vi "CalGas Filtern - Elemente ermitteln.vi"(8 "über GT":bool, 9 "CalGase":u16[](array[numeric]), 10 "MB KAL":u16[](array[numeric]), 11 "derzeitiger Messbereich":i32) -> (0 "Einheit":T3, 1 "Messberich":T3, 2 "Wert 2":T11 format="%#_5g", 3 "Wert 1":T11 format="%#_5g", 4 "OK":bool, 5 "Name":T3, 6 "CalGas":i32, 7 "Messbereich":u16)   [LabVIEW 2020, in "CalGas Aufschaltung.lvlib"]
uses:
  CalGas Aufschaltung.lvlib
  Visualisierungs Elemente/Zahlen-Ausgabefeld.ctl
  Visualisierungs Elemente/String - Ausgabefeld.ctl
  Definition CalGas Anzeige.ctl
  CalGas-Namen.ctl
  Visualisierungs Elemente/String - Eingabefeld.ctl
  CalGas-Werte.ctl
  Visualisierungs Elemente/Zahlen-Eingabefeld.ctl
  CalGas-Einheit.ctl
  Visualisierungs Elemente/Auswahlfeld.ctl
  CalGas-Messbereiche.ctl
  Aufschaltung CalGas_ANZEIGE.ctl
  FGV CalGas Aktionen.ctl
  Linearisierung V2/Aktion Lin Daten aufarbeiten.ctl
  Analysator Definition/FGV Analysator Definition Aktionen.ctl
  Linearisierung V2/Linearisierung v2.lvlib
  Analysator Definition/Analysator Definition.lvlib
panel:
  in  "Aufschaltung CalGas":T1 {"Analysator" items=["FT-IR", "FID", "PMD", "PMD/FID/FT-IR"]; "Aufschaltpunkt" items=["Filterblock", "Analyzer directly", "PNS"]; "Kalibriergas" items=["Stickstoff", "", "FID SPAN", "Gasteiler", "O2", "", "", "", "", "", "", "", ""]}
  in  "Def.CalGas":T4 {"Messbereiche"."Messbereich 12" items=["0-100ppm", "0-1000ppm", "0-5000ppm"]; "Messbereiche"."Messbereich 11" items=["0-100ppm", "0-1000ppm", "0-5000ppm"]; "Messbereiche"."Messbereich 10" items=["0-100ppm", "0-1000ppm", "0-5000ppm"]; "Messbereiche"."Messbereich 9" items=["0-100ppm", "0-1000ppm", "0-5000ppm"]; "Messbereiche"."Messbereich 8" items=["0-100ppm", "0-1000ppm", "0-5000ppm"]; "Messbereiche"."Messbereich 7" items=["0-100ppm", "0-1000ppm", "0-5000ppm"]; "Messbereiche"."Messbereich 6" items=["0-100ppm", "0-1000ppm", "0-5000ppm"]; "Messbereiche"."Messbereich 5" items=["0-100ppm", "0-1000ppm", "0-5000ppm"]; "Messbereiche"."Messbereich 4" items=["0-100ppm", "0-1000ppm", "0-5000ppm"]; "Messbereiche"."Messbereich 3" items=["0-100ppm", "0-1000ppm", "0-5000ppm"]; "Messbereiche"."Messbereich 2" items=["0-100ppm", "0-1000ppm", "0-5000ppm"]; "Messbereiche"."Messbereich 1" items=["0-100ppm", "0-1000ppm", "0-5000ppm"]; "Einheit"."Einheit 12" items=["ppm", "%"]; "Einheit"."Einheit 11" items=["ppm", "%"]; "Einheit"."Einheit 10" items=["ppm", "%"]; "Einheit"."Einheit 9" items=["ppm", "%"]; "Einheit"."Einheit 8" items=["ppm", "%"]; "Einheit"."Einheit 7" items=["ppm", "%"]; "Einheit"."Einheit 6" items=["ppm", "%"]; "Einheit"."Einheit 5" items=["ppm", "%"]; "Einheit"."Einheit 4" items=["ppm", "%"]; "Einheit"."Einheit 3" items=["ppm", "%"]; "Einheit"."Einheit 2" items=["ppm", "%"]; "Einheit"."Einheit 1" items=["ppm", "%"]; "Werte 2"."Konzentration 12" format="%#_5g"; "Werte 2"."Konzentration 11" format="%#_5g"; "Werte 2"."Konzentration 10" format="%#_5g"; "Werte 2"."Konzentration 9" format="%#_5g"; "Werte 2"."Konzentration 8" format="%#_5g"; "Werte 2"."Konzentration 7" format="%#_5g"; "Werte 2"."Konzentration 6" format="%#_5g"; "Werte 2"."Konzentration 5" format="%#_5g"; "Werte 2"."Konzentration 4" format="%#_5g"; "Werte 2"."Konzentration 3" format="%#_5g"; "Werte 2"."Konzentration 2" format="%#_5g"; "Werte 2"."Konzentration 1" format="%#_5g"; "Werte"."Konzentration 12" format="%#_5g"; "Werte"."Konzentration 11" format="%#_5g"; "Werte"."Konzentration 10" format="%#_5g"; "Werte"."Konzentration 9" format="%#_5g"; "Werte"."Konzentration 8" format="%#_5g"; "Werte"."Konzentration 7" format="%#_5g"; "Werte"."Konzentration 6" format="%#_5g"; "Werte"."Konzentration 5" format="%#_5g"; "Werte"."Konzentration 4" format="%#_5g"; "Werte"."Konzentration 3" format="%#_5g"; "Werte"."Konzentration 2" format="%#_5g"; "Werte"."Konzentration 1" format="%#_5g"}
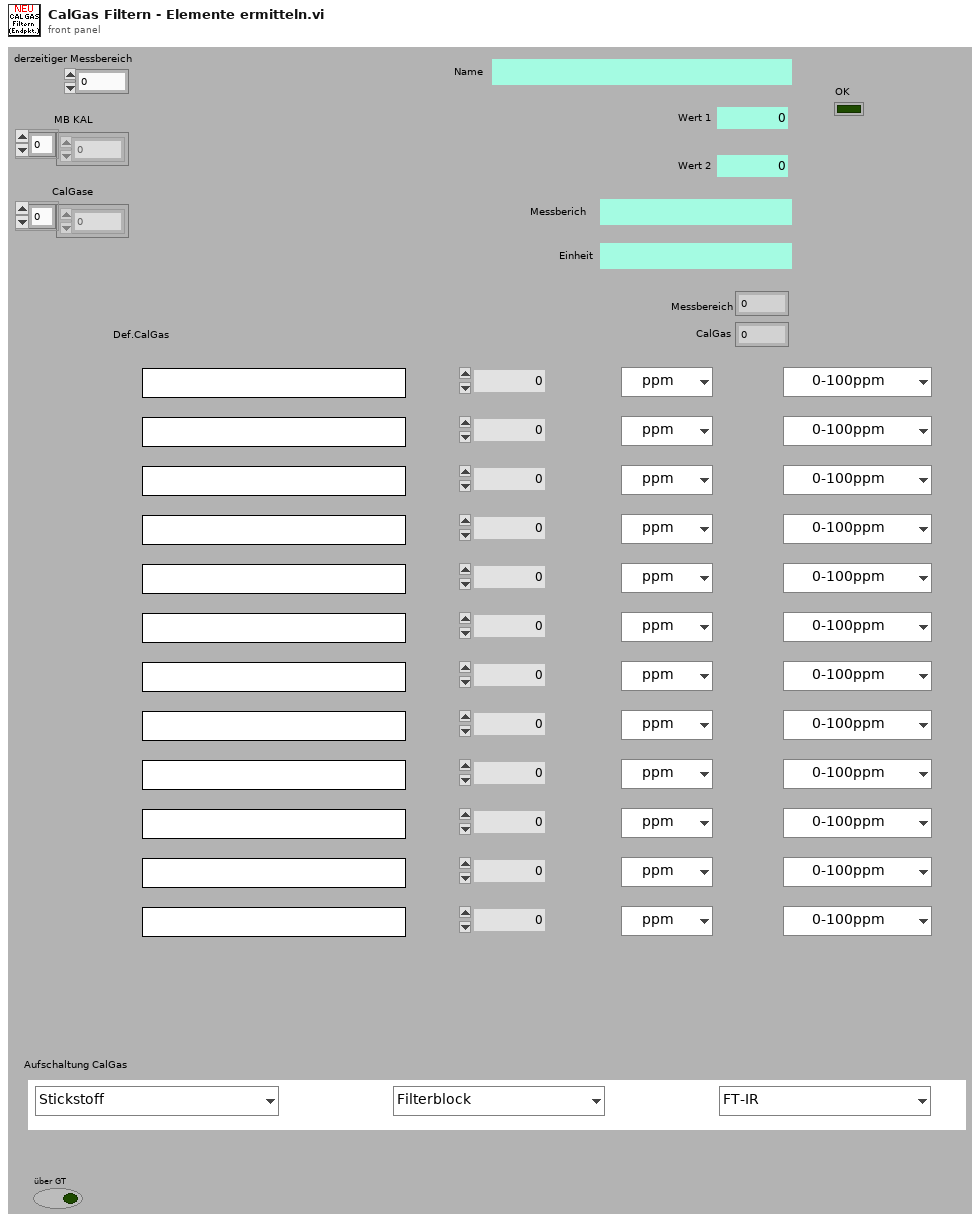
[diagram p1: front panel]
types:
  T1 = typedef "CalGas Aufschaltung.lvlib/Aufschaltung CalGas_ANZEIGE.ctl" = cluster{"Kalibriergas":T2, "Aufschaltpunkt":T2, "Analysator":T2}
  T2 = typedef "Auswahlfeld.ctl" = u16
  T3 = typedef "String - Ausgabefeld.ctl" = string
  T4 = typedef "CalGas Aufschaltung.lvlib/Definition CalGas Anzeige.ctl" = cluster{"Namen":T5, "Werte":T7, "Werte 2":T7, "Einheit":T9, "Messbereiche":T10}
  T5 = typedef "CalGas Aufschaltung.lvlib/CalGas-Namen.ctl" = cluster{"Name":T6, "Name 2":T6, "Name 3":T6, "Name 4":T6, "Name 5":T6, "Name 6":T6, "Name 7":T6, "Name 8":T6, "Name 9":T6, "Name 10":T6, "Name 11":T6, "Name 12":T6}
  T6 = typedef "String - Eingabefeld.ctl" = string
  T7 = typedef "CalGas Aufschaltung.lvlib/CalGas-Werte.ctl" = cluster{"Konzentration 1":T8, "Konzentration 2":T8, "Konzentration 3":T8, "Konzentration 4":T8, "Konzentration 5":T8, "Konzentration 6":T8, "Konzentration 7":T8, "Konzentration 8":T8, "Konzentration 9":T8, "Konzentration 10":T8, "Konzentration 11":T8, "Konzentration 12":T8}
  T8 = typedef "Zahlen-Eingabefeld.ctl" = sgl
  T9 = typedef "CalGas Aufschaltung.lvlib/CalGas-Einheit.ctl" = cluster{"Einheit 1":T2, "Einheit 2":T2, "Einheit 3":T2, "Einheit 4":T2, "Einheit 5":T2, "Einheit 6":T2, "Einheit 7":T2, "Einheit 8":T2, "Einheit 9":T2, "Einheit 10":T2, "Einheit 11":T2, "Einheit 12":T2}
  T10 = typedef "CalGas Aufschaltung.lvlib/CalGas-Messbereiche.ctl" = cluster{"Messbereich 1":T2, "Messbereich 2":T2, "Messbereich 3":T2, "Messbereich 4":T2, "Messbereich 5":T2, "Messbereich 6":T2, "Messbereich 7":T2, "Messbereich 8":T2, "Messbereich 9":T2, "Messbereich 10":T2, "Messbereich 11":T2, "Messbereich 12":T2}
  T11 = typedef "Zahlen-Ausgabefeld.ctl" = sgl
  T12 = typedef "CalGas Aufschaltung.lvlib/FGV CalGas Aktionen.ctl" = enum16{"lesen", "Analysator Auswahl", "Def.CalGas", "Aufschaltung CalGas", "laden", "speichern", "KAL extrahieren"}
  T13 = typedef "Analysator Definition.lvlib/FGV Analysator Definition Aktionen.ctl" = enum16{"lesen", "MB setzen", "MB KAL setzen", "laden"}
  T14 = typedef "Linearisierung v2.lvlib/Aktion Lin Daten aufarbeiten.ctl" = enum16{"lesen", "Protkolldaten", "speichern", "laden", "EPA auswerten", "Tabelle schreiben", "Lin auswerten", "Tab init", "Stufentabelle", "EPA aktiviert", "Nachbehandlung laden", "Tabelle löschen", "Istwerte löschen", "Zeile löschen", "Zeile einfügen", "LIN aktiviert", "LIN/EPA aktiv laden", "EGAK Tab", "LIN übernehmen", "Tab init ohne Stufen"}
  T15 = typedef "CalGas Aufschaltung.lvlib/Aufschaltung CalGas.ctl" = cluster{"Kalibriergas":T2, "Aufschaltpunkt":T16, "Analysator":T17}
  T16 = typedef "CalGas Aufschaltung.lvlib/Auswahl Aufschaltpunkt.ctl" = enum16{"über Filterblock", "Analysator direkt", "über PNS", "Entnahme", "Gasdivider"}
  T17 = typedef "CalGas Aufschaltung.lvlib/Auswahl Analysator.ctl" = enum16{"FT-IR", "FID", "PMA", "PMA/FID/FT-IR"}
  T18 = typedef "Linearisierung v2.lvlib/Lin-Polynom Daten.ctl" = cluster{"Messgerät":string, "Kalibrator (Gasteiler)":string, "Bearbeiter/in":string, "Komponente":string, "Zeitstempel":timestamp, "F_max gefordert (%)":sgl, "F_max in %":sgl, "F_max in ppm":sgl, "Vorschlag Ordnung":i32, "Polynom OK":bool, "Polynomkoeff.":dbl[], "Prüfgas Konzentration":dbl, "Pfad EPA":string, "Pfad_LIN":string, "Gasnummer:":u8, "Komponentenauswahl":T19, "Verdünnungsgas":T20, "Zeitdauer Stufe":T8, "Anzahl Stufen":T8, "F_max in % EPA":sgl, "F_max in ppm EPA":sgl, "F_max in % LIN":sgl, "F_max in ppm LIN":sgl, "Punkte umkehren":bool, "EPA Optionsfeld":T21, "Autolin Hovacal":T22, "Spanfactors":sgl[], "Kalibrierauswahl":T23, "Conditions:":T24, "Gasflaschen Nr.:":string, "Bottle Accuracy":dbl, "Konfig Gasflasche":T25, "Gasflasche":T26, "HovaCAL Flow AutoLin":T27, "MFC Output":T28, "Gas Ablaufdatum":timestamp, "Lin Modus":T29, "zusätzliche Zeitdauer Erster Punkt":sgl, "Offsets":sgl[]}
  T19 = typedef "Linearisierung v2.lvlib/KomponentenArray.ctl" = cluster{"Komponente:":T2, "Konzentration":dbl}[]
  T20 = typedef "Linearisierung v2.lvlib/Gasteiler.lvlib/Prüfgas in.ctl" = u16
  T21 = typedef "Linearisierung v2.lvlib/EPA Optionsfeld.ctl" = enum32{"Istwert", "Rohwert", "Linearisierter Wert"}
  T22 = typedef "Linearisierung v2.lvlib/Gasteiler.lvlib/HovaCal.lvlib/AutoLin Hovacal.ctl" = enum32{"Keine Auswahl", "Optionsauswahl 1", "Optionsauswahl 2"}
  T23 = typedef "Linearisierung v2.lvlib/Kalibrieroption.ctl" = u16
  T24 = typedef "Linearisierung v2.lvlib/Linearity verification 1065-307.lvlib/Condition.ctl" = u16
  T25 = typedef "System Einstellungen V2.lvlib/Konfig Gasflasche.ctl" = bool
  T26 = typedef "System Einstellungen V2.lvlib/Gasflasche Auswahl.ctl" = u16
  T27 = typedef "Linearisierung v2.lvlib/Gasteiler.lvlib/HovaCAL_Interface.lvlib/Controls.lvlib/Flow Einstellung.ctl" = cluster{"HovaCAL Flow Input Cluster":dbl}
  T28 = typedef "Linearisierung v2.lvlib/Gasteiler.lvlib/HovaCAL_Interface.lvlib/Controls.lvlib/Pump state.ctl" = cluster{"Run":bool}
  T29 = typedef "CalGas Aufschaltung.lvlib/Lin Modus.ctl" = u16
  T30 = typedef "Analysator Definition.lvlib/Betriebsdaten Komponente.ctl" = cluster{"Namen":string[], "MB Namen":string[], "Einheit":string, "MB Aktuell":u16, "MB Endwert":u16, "CalGase":u16[], "MB für KAL":u16[], "CG für KAL":u16[]}
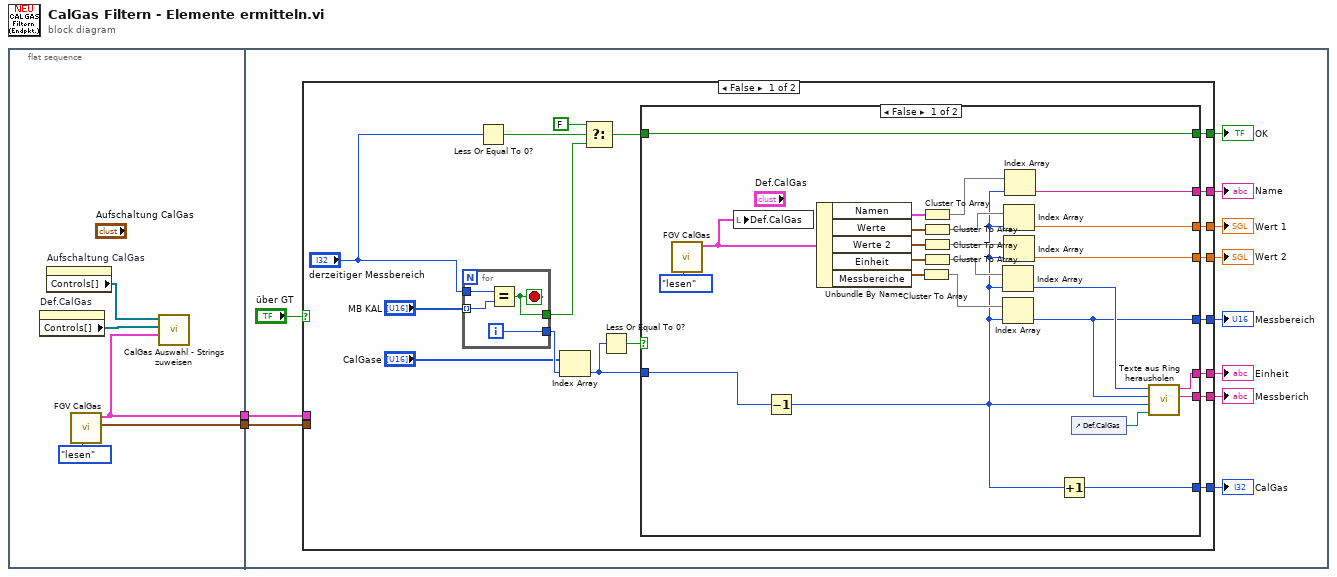
[diagram p0: block diagram]
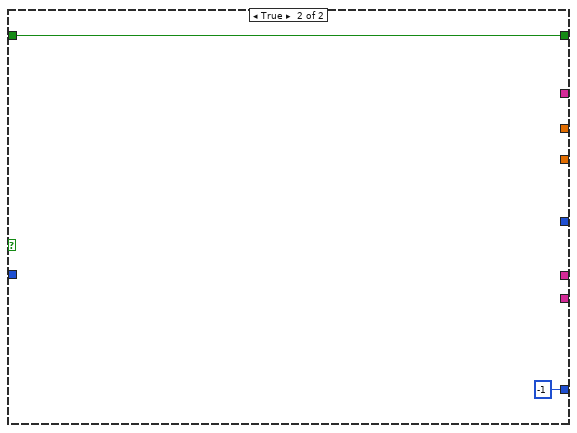
[diagram p2: hidden frame]
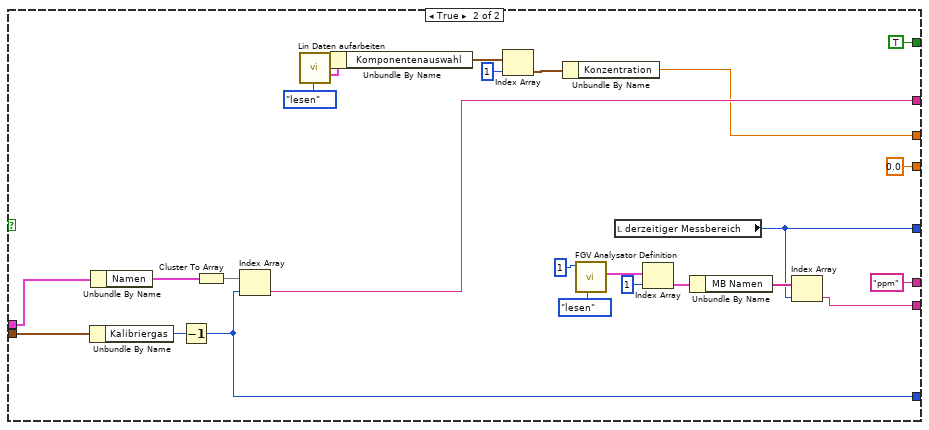
[diagram p3: hidden frame]
diagram:
  n1 = flat-sequence {
    tunnel: [w4] -> w2
    tunnel: [w3] -> w1
    tunnel: w2 -> [w9]
    tunnel: w1 -> [w8]
    frame #0 {
      n2 = property on="Def.CalGas" class="Cluster (strikt)"() -> ("Controls[]"=w7:refnum<vi>[])  [unwired: 2 in, 2 out]
      n3 = property on="Aufschaltung CalGas" class="Cluster (strikt)"() -> ("Controls[]"=w6:refnum<vi>[])  [unwired: 2 in, 2 out]
      n4 = call "FGV CalGas.vi"("Aktionen"=FGV_CalGas_Aktionen."lesen") -> ("Aufschaltung CalGas"=w4:T15, "Def.CalGas"=w3:T4)  [unwired: 6 in, 3 out]
      n5 = call "CalGas Auswahl - Strings zuweisen.vi"(9:"Def.CalGas"=w3, 10:"Def.CalGas"=w7, "Aufschaltung CalGas"=w6) -> ()  [unwired: 8 in, 1 out]
    }
    frame #1 {
      n6 = case shown="False" "über GT" {
        tunnel: [w36 T3 "ppm" ("Einheit")] -> w18
        tunnel: [w35 w67] -> w17
        tunnel: [w34 w83] -> w16
        tunnel: [w33 w77] -> w15
        tunnel: [w32 T8 0.0 ("Konzentration 1")] -> w14
        tunnel: [w31 w68] -> w13
        tunnel: [w30 w76] -> w12
        tunnel: [w25 TRUE ("t")] -> w11
        tunnel: w9 -> [_ w90]
        tunnel: w8 -> [_ w88]
        frame False {
          n7 = for {
            tunnel: "derzeitiger Messbereich" -> [w39]
            tunnel: "MB KAL" -> [w40] mode=indexing
            tunnel: [w38] -> w29
            tunnel: [w37] -> w23
            i -> [w38]
            stop <- w37 stop-if-true
            n8 = Equal?(x=w39, y=w40) -> (x = y?=w37:bool)
          }
          n9 = Less Or Equal To 0?(x="derzeitiger Messbereich") -> (x <= 0?=w24:bool)
          n10 = Index Array(array="CalGase", index=w29) -> (element=w28:u16)
          n11 = Select(t=FALSE, s=w24, f=w23) -> (s? t:f=w21:bool)
          n12 = Less Or Equal To 0?(x=w28) -> (x <= 0?=w26:bool)
          n13 = case shown="False" w26 {
            tunnel: [w52 _] -> w36
            tunnel: [w50 _] -> w35
            tunnel: [w49 _] -> w34
            tunnel: [w48 _] -> w33
            tunnel: [w47 _] -> w32
            tunnel: [w41 _] -> w31
            tunnel: [w45 -1] -> w30
            tunnel: w28 -> [w44 _]
            tunnel: w21 -> [w43 w65]
            tunnel: [w43 w65] -> w25
            frame False {
              n14 = call "FGV CalGas.vi"("Aktionen"=FGV_CalGas_Aktionen."lesen") -> ("Def.CalGas"=w42:T4)  [unwired: 6 in, 4 out]
              n15 = local write "Def.CalGas"(w42) -> ()
              n16 = Decrement(x=w44) -> (x-1=w46:u16)
              n17 = Unbundle By Name(w42) -> ("Namen"=w63:T5, "Werte"=w62:T7, "Werte 2"=w61:T7, "Einheit"=w60:T9, "Messbereiche"=w55:T10)
              n18 = Cluster To Array(cluster=w55) -> (array=w54:T2[])
              n19 = Cluster To Array(cluster=w63) -> (array=w59:T6[])
              n20 = Cluster To Array(cluster=w62) -> (array=w58:T8[])
              n21 = Cluster To Array(cluster=w61) -> (array=w57:T8[])
              n22 = Cluster To Array(cluster=w60) -> (array=w56:T2[])
              n23 = Index Array(array=w56, index=w46) -> (element=w51:T2)
              n24 = Index Array(array=w54, index=w46) -> (element=w41:T2)
              n25 = Index Array(array=w58, index=w46) -> (element=w48:T8)
              n26 = Index Array(array=w57, index=w46) -> (element=w47:T8)
              n27 = Index Array(array=w59, index=w46) -> (element=w49:T6)
              n28 = Increment(x=w46) -> (x+1=w45:u16)
              n29 = control-ref of="Def.CalGas"() -> (w53:refnum<vi>)
              n30 = call "Texte aus Ring herausholen.vi"("Def.CalGas"=w53, "Gas"=w46, "Element Messbereich"=w41, "Element Einheit"=w51) -> ("Messberich"=w50:T3, "Einheit"=w52:T3)  [unwired: 6 in]
            }
            frame True {
            }
          }
        }
        frame True {
          n31 = Unbundle By Name(w90) -> ("Kalibriergas"=w84:T2)
          n32 = Unbundle By Name(w88) -> ("Namen"=w85:T5)
          n33 = Decrement(x=w84) -> (x-1=w76:T2)
          n34 = Cluster To Array(cluster=w85) -> (array=w86:T6[])
          n35 = Index Array(array=w86, index=w76) -> (element=w83:T6)
          n36 = call "Lin Daten aufarbeiten.vi"("Aktionen"=Aktion_Lin_Daten_aufarbeiten."lesen") -> ("Lin-Polynom"=w81:T18)  [unwired: 16 in, 10 out]
          n37 = Unbundle By Name(w81) -> ("Komponentenauswahl"=w80:T19)
          n38 = Index Array(array=w80, index=1 ("Index")) -> (element=w78:cluster{"Komponente:":T2, "Konzentration":dbl})
          n39 = Unbundle By Name(w78) -> ("Konzentration"=w77:dbl)
          n40 = call "FGV Analysator Definition.vi"("Aktionen"=FGV_Analysator_Definition_Aktionen."lesen", "Komponente"=1) -> ("Betriebsdaten"=w72:T30[])  [unwired: 5 in, 4 out]
          n41 = local read "derzeitiger Messbereich"() -> (w68:i32)
          n42 = Index Array(array=w72, index=1 ("Index")) -> (element=w70:T30)
          n43 = Unbundle By Name(w70) -> ("MB Namen"=w69:string[])
          n44 = Index Array(array=w69, index=w68) -> (element=w67:string)
        }
      }
      "Wert 1" <- w15
      "Name" <- w16
      "Wert 2" <- w14
      "Messberich" <- w17
      "Einheit" <- w18
      "Messbereich" <- w13
      "CalGas" <- w12
      "OK" <- w11
    }
  }
